vi "MVC.vi"() -> (8 "mean":dbl=4.09184727350889 format="%0.2f")   [LabVIEW 2011]
uses:
  <vilib>/Analysis/NI_AAL_SigProc.lvlib
  <vilib>/Analysis/NI_AALBase.lvlib
panel:
  out "Amplitudes":dbl[](array[numeric])=[3.9040889326746515, 4.8149945507435445, 3.5564583371084733]
  in  "Filename":path=path "C:/Users/Sinha/Desktop/Ankle/MaxMC/test.csv"
  in  "threshold":dbl=0.6
  out "# found":i32=3
  out "Waveform Chart":dbl[][](graph)=[[-0.21484375, 0.7], [-0.21484375, 0.7], [-0.21240234375, 0.7], [-0.21484375, 0.7], [-0.21484375, 0.7], [-0.21484375, 0.7], [-0.21484375, 0.7], [-0.21484375, 0.7], [-0.21240234375, 0.7], [-0.21484375, 0.7]]
  in  "stop (F)":bool
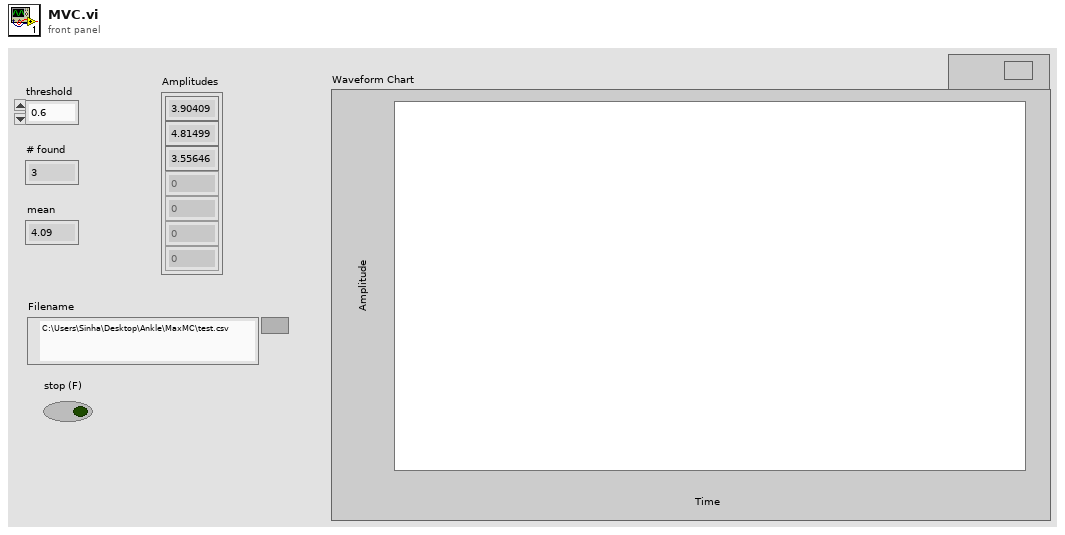
[diagram p1: front panel]
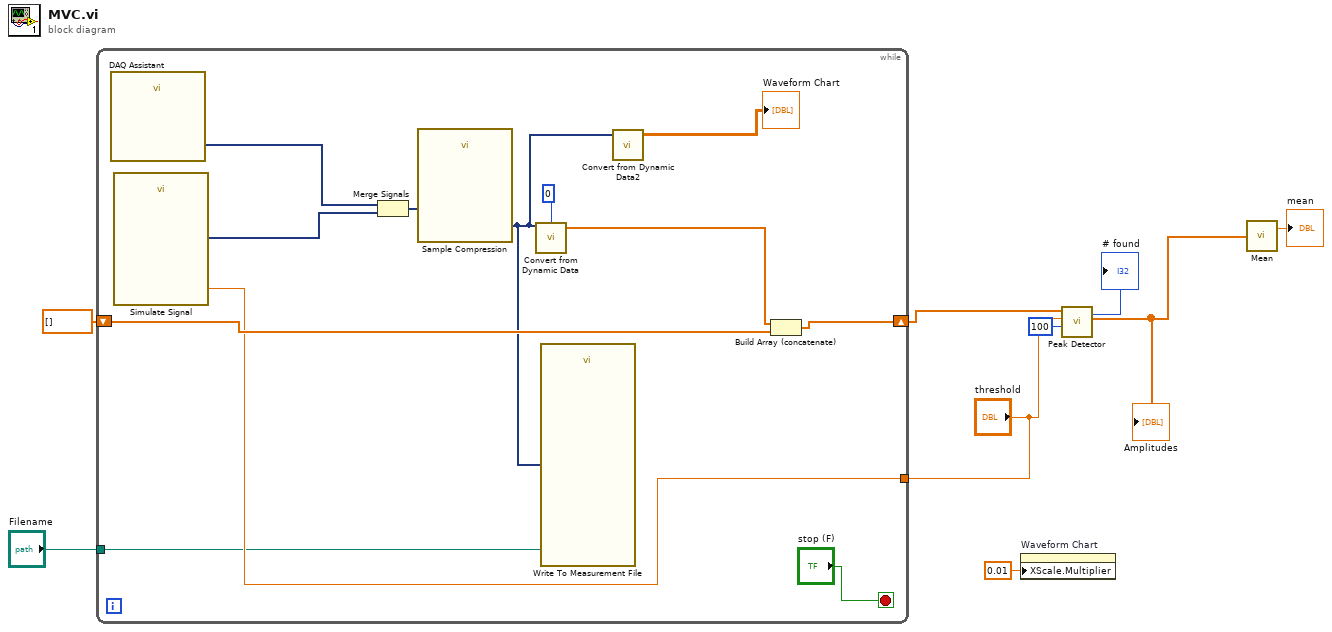
[diagram p0: block diagram]
diagram:
  n1 = while {
    shift-right: [w19] -> w8
    shift-left: dbl[] [] -> [w20]
    tunnel: "threshold" -> [w16]
    tunnel: "Filename" -> [w10]
    stop <- "stop (F)" stop-if-true
    n2 = call "DAQ Assistant"() -> ("data"=w15:dynamicdata)  [unwired: 16 in, 3 out]
    n3 = call "Simulate Signal"("Offset"=w16) -> ("DC"=w18:dynamicdata)  [unwired: 13 in, 1 out]
    n4 = Merge Signals(w15, w18) -> (w14:dynamicdata)
    n5 = call "Sample Compression"("Signals"=w14) -> ("Median"=w11:dynamicdata)  [unwired: 8 in, 2 out]
    n6 = call "Convert from Dynamic Data"("Dynamic Data Type"=w11, "Channel"=0) -> ("Array"=w21:dbl[])  [unwired: 2 in]
    n7 = call "Write To Measurement File"("Signals"=w11, "Filename"=w10) -> ()  [unwired: 15 in, 3 out]
    n8 = call "Convert from Dynamic Data2"("Dynamic Data Type"=w11) -> ("Array"=→"Waveform Chart":dbl[][])  [unwired: 3 in]
    n9 = Build Array (concatenate)(w21, w20) -> (w19:dbl[])
  }
  n10 = property on="Waveform Chart" class="WFChart (strict)"("XScale.Multiplier"=0.01 ("X Scale.Offset and Multiplier:Multiplier")) -> ()  [unwired: 2 in, 2 out]
  n11 = call <vilib>:"Peak Detector.vi"("width"=100, "threshold"="threshold", "X"=w8) -> ("Amplitudes"=w3:dbl[], "# found"=→"# found":i32)  [unwired: 4 in, 3 out]
  "Amplitudes" <- w3
  n12 = call <vilib>:"Mean.vi"("X"=w3) -> ("mean"=→"mean":dbl)  [unwired: 1 out]
